vi "提取经纬度.vi"(11 "body":string) -> (2 "纬度":string, 3 "经度":string)   [LabVIEW 2015]
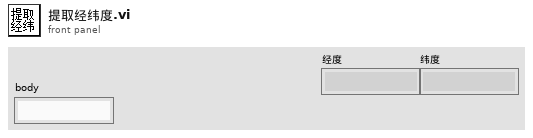
[diagram p1: front panel]
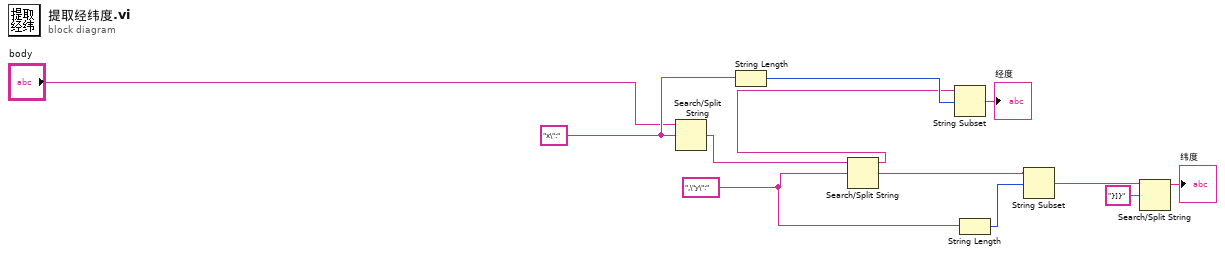
[diagram p0: block diagram]
diagram:
  w8 = ",\"y\":" ("搜索字符串/字符(-)")
  w4 = "x\":" ("搜索字符串/字符(-)")
  n1 = Search/Split String(string="body", search string/char (-)=w4) -> (match + rest of string=w5:string)  [unwired: 1 in, 2 out]
  n2 = String Length(string=w4) -> (length=w7:i32)
  n3 = Search/Split String(string=w5, search string/char (-)=w8) -> (substring before match=w6:string, match + rest of string=w9:string)  [unwired: 1 in, 1 out]
  n4 = String Subset(string=w6, offset (0)=w7) -> (substring=→"经度":string)  [unwired: 1 in]
  n5 = String Length(string=w8) -> (length=w10:i32)
  n6 = String Subset(string=w9, offset (0)=w10) -> (substring=w11:string)  [unwired: 1 in]
  n7 = Search/Split String(string=w11, search string/char (-)="}]}" ("搜索字符串/字符(-)")) -> (substring before match=→"纬度":string)  [unwired: 1 in, 2 out]
